vi "WS1021 MEMS Only CS Data Convert.vi"(8 "Error In":errorcluster, 11 "Data In":string[][](array[string])) -> (0 "Error Out":errorcluster, 1 "V3":string[][](array[string]), 2 "V2":string[][](array[string]), 3 "V1":string[][](array[string]), 5 "Data Out":string[][](array[string]))   [LabVIEW 2017]
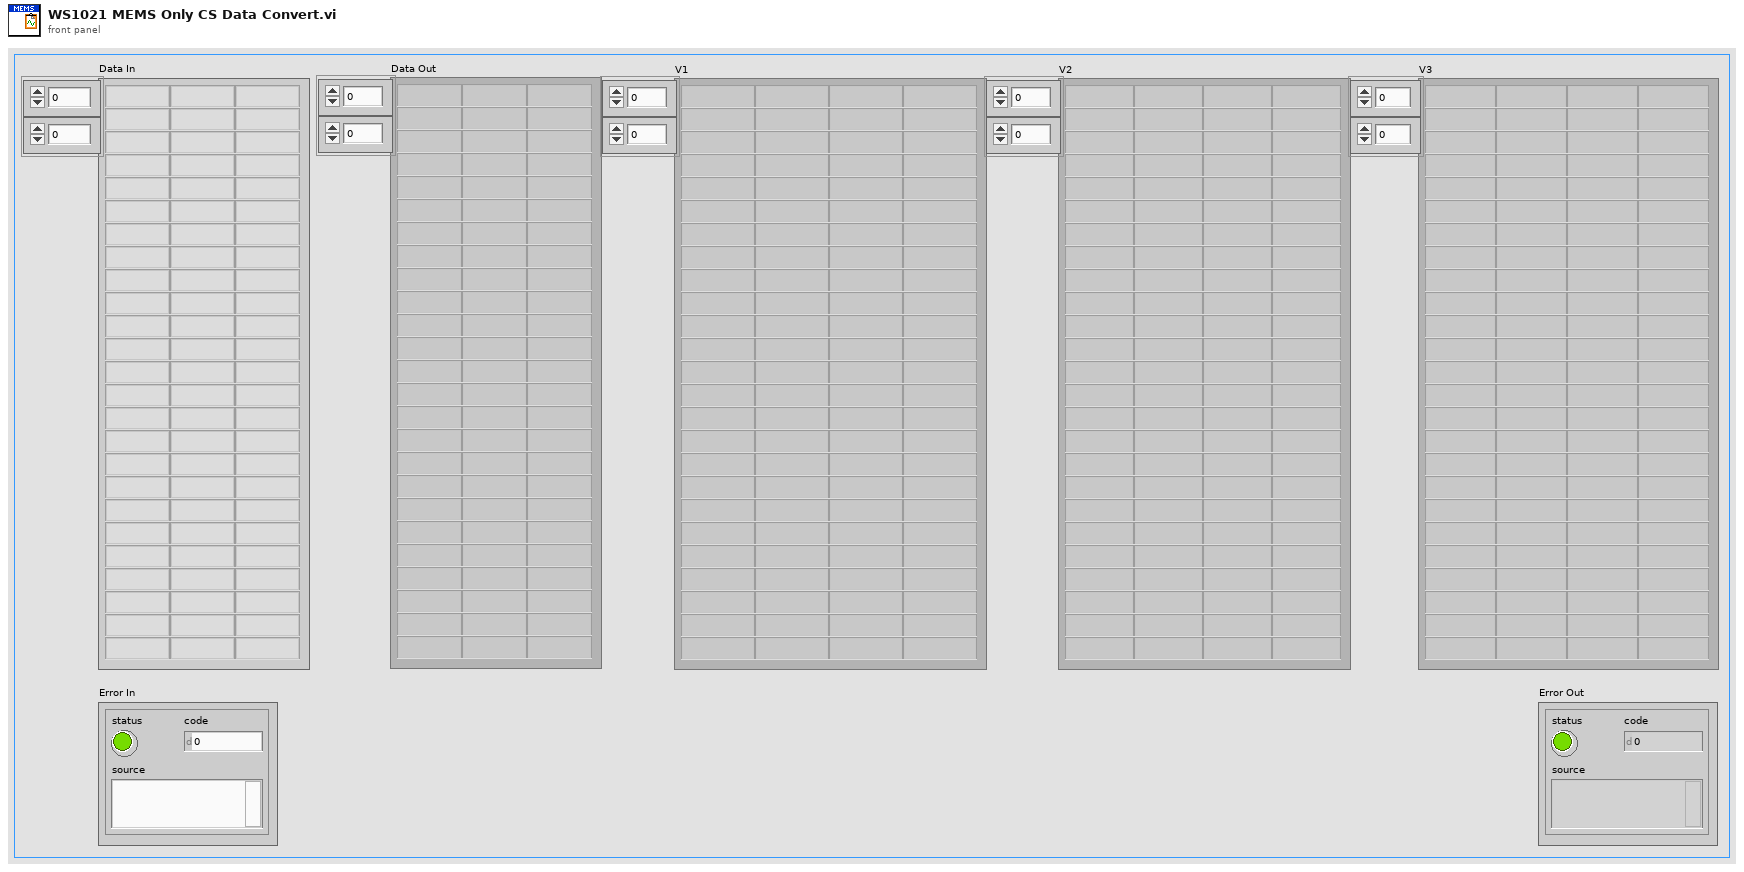
[diagram p1: front panel]
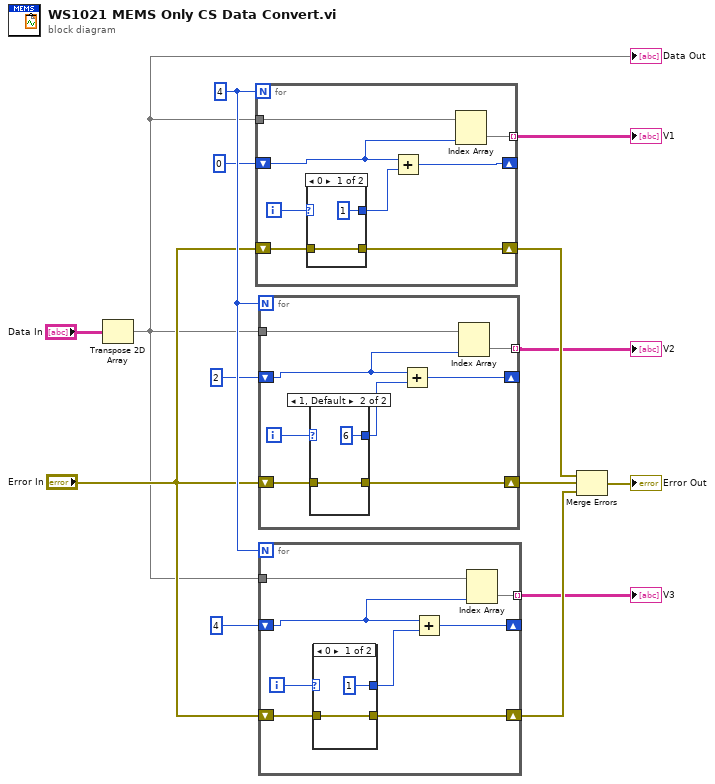
[diagram p0: block diagram]
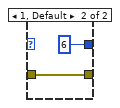
[diagram p2: hidden frame]
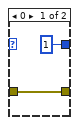
[diagram p3: hidden frame]
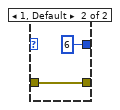
[diagram p4: hidden frame]
diagram:
  w14 = 4
  n1 = Transpose 2D Array(2D array="Data In") -> (transposed array=w4:string[][])
  "Data Out" <- w4
  n2 = for {
    N: w14 -> [_]
    tunnel: w4 -> [w22]
    tunnel: [w20] -> w1 mode=indexing
    shift-right: [w18] -> _
    shift-left: 0 -> [w17]
    shift-right: [w15] -> w8
    shift-left: "Error In" -> [w16]
    i -> [w21]
    n3 = case shown="0" w21 {
      tunnel: [1 6] -> w19
      tunnel: w16 -> [w23 w25]
      tunnel: [w23 w25] -> w15
      frame 0 {
      }
      frame 1, Default {
      }
    }
    n4 = Add(x=w17, y=w19) -> (x+y=w18:i32)
    n5 = Index Array(array=w22, index (col)=w17) -> (element=w20:string[])  [unwired: 1 in]
  }
  "V1" <- w1
  n6 = for {
    N: w14 -> [_]
    tunnel: w4 -> [w34]
    tunnel: [w32] -> w2 mode=indexing
    shift-right: [w30] -> _
    shift-left: 2 -> [w29]
    shift-right: [w27] -> w9
    shift-left: "Error In" -> [w28]
    i -> [w33]
    n7 = case shown="1, Default" w33 {
      tunnel: [1 6] -> w31
      tunnel: w28 -> [w35 w37]
      tunnel: [w35 w37] -> w27
      frame 0 {
      }
      frame 1, Default {
      }
    }
    n8 = Add(x=w29, y=w31) -> (x+y=w30:i32)
    n9 = Index Array(array=w34, index (col)=w29) -> (element=w32:string[])  [unwired: 1 in]
  }
  "V2" <- w2
  n10 = for {
    N: w14 -> [_]
    tunnel: w4 -> [w46]
    tunnel: [w44] -> w3 mode=indexing
    shift-right: [w42] -> _
    shift-left: 4 -> [w41]
    shift-right: [w39] -> w7
    shift-left: "Error In" -> [w40]
    i -> [w45]
    n11 = case shown="0" w45 {
      tunnel: [1 6] -> w43
      tunnel: [w47 w49] -> w39
      tunnel: w40 -> [w47 w49]
      frame 0 {
      }
      frame 1, Default {
      }
    }
    n12 = Add(x=w41, y=w43) -> (x+y=w42:i32)
    n13 = Index Array(array=w46, index (col)=w41) -> (element=w44:string[])  [unwired: 1 in]
  }
  "V3" <- w3
  n14 = Merge Errors(w8, w9, w7) -> (→"Error Out":errorcluster)
